vi "LVClass_CorrectionDataManager SetPupilMask.vi"(0 "CorrectionDataManager in":refnum<class "CorrectionDataManager.lvclass">, 5 "Pupil in":refnum<class "Pupil.lvclass">, 11 "error in (no error)":errorcluster) -> (4 "CorrectionDataManager out":refnum<class "CorrectionDataManager.lvclass">, 6 "Pupil out":refnum<class "Pupil.lvclass">, 15 "error out":errorcluster)   [LabVIEW 2020, in "CorrectionDataManager.lvclass"]
doc: "Modifies the greatest common pupil.\n\n<B>corrdata_managerIn</B> : CorrDataManager object.\n<B>corrdata_managerOut</B> : CorrDataManager object.\n<B>pupil_mask</B> : User-defined pupil mask as a pointer on a pupil object."
uses:
  CorrectionDataManager.lvclass
  Pupil/Pupil.lvclass
  Pupil/LVClass_Pupil Read Pupil.vi
  LVClass_CorrectionDataManager Read CorrectionDataManager.vi
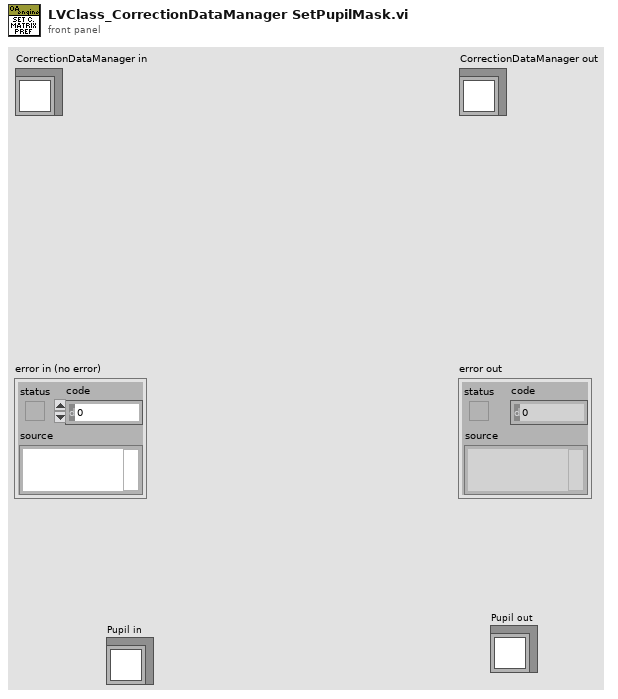
[diagram p1: front panel]
types:
  T1 = typedef "ClassID.ctl" = i64
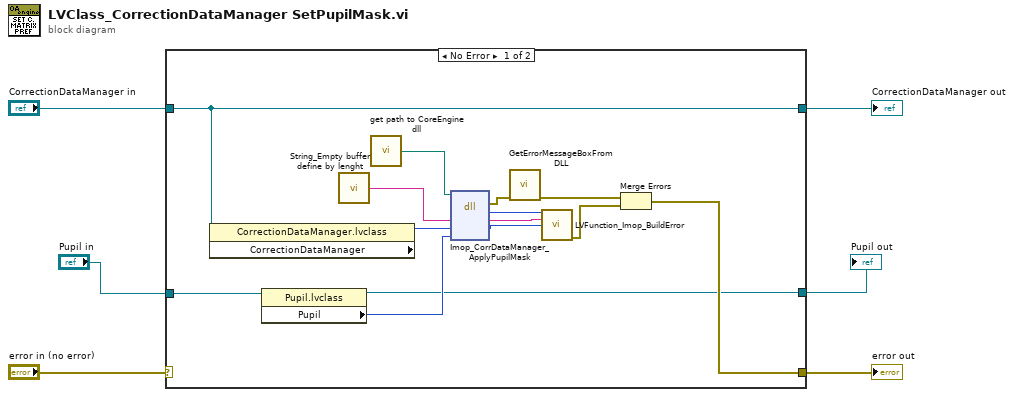
[diagram p0: block diagram]
diagram:
  n1 = case shown="No Error" "error in (no error)" {
    selector: "error in (no error)" -> [_ w23]
    tunnel: [w12 w23] -> w5
    tunnel: [w13 w22] -> w6
    tunnel: "CorrectionDataManager in" -> [w13 w22]
    tunnel: "Pupil in" -> [w10 w21]
    tunnel: [w8 w21] -> w1
    frame No Error {
      n2 = property class="CorrectionDataManager.lvclass"(reference=w13) -> ("CorrectionDataManager"=w11:T1)  [unwired: 1 in, 2 out]
      n3 = property class="Pupil.lvclass"(reference=w10) -> (reference out=w8:refnum<class "Pupil.lvclass">, "Pupil"=w9:T1)  [unwired: 1 in, 1 out]
      n4 = call "String_Empty buffer define by lenght.vi"() -> ("Empty buffer"=w18:string)  [unwired: 1 in]
      n5 = call "get path to CoreEngine dll.vi"() -> ("path to wavekit library"=w17:path)  [unwired: 14 in, 1 out]
      n6 = dll-call lib="D:/soft/HASO_v3/SVN_trunk/ImOpCoreEngine4_LV2011/DLLs/c_interface_vc100.dll" fn="Imop_CorrDataManager_ApplyPupilMask"(path in=w17, "message"=w18, "WavefrontCorrection"=w11, "pupil"=w9) -> (error out=w16:errorcluster, "return type"=w20:i32, "message"=w19:string, "WavefrontCorrection"=w7:i64)  [unwired: 3 in, 1 out]
      n7 = call "GetErrorMessageBoxFromDLL.vi"("error IN"=w16) -> ("error OUT"=w15:errorcluster)  [unwired: 10 in]
      n8 = call "LVFunction_Imop_BuildError.vi"("code"=w20, "String to Prepend to source (\"\")"=w19, "Adresse"=w7) -> ("error out"=w14:errorcluster)  [unwired: 12 in]
      n9 = Merge Errors(w15, w14) -> (w12:errorcluster)
    }
    frame Error {
    }
  }
  "error out" <- w5
  "CorrectionDataManager out" <- w6
  "Pupil out" <- w1
